vi "Send Message_test.vi"(2 "msj":string, 4 "error in (no error)":errorcluster, 5 "Process":i32, 6 "List of process":string[][](array[string]), 7 "Send msj":bool) -> (0 "error out":errorcluster)   [LabVIEW 2022 SP3]
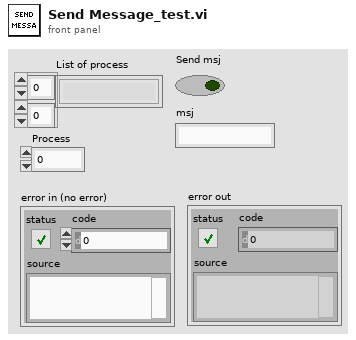
[diagram p1: front panel]
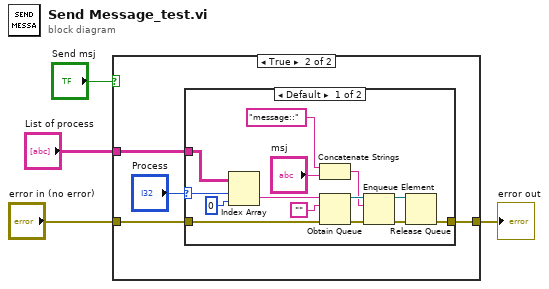
[diagram p0: block diagram]
diagram:
  n1 = case shown="True" "Send msj" {
    tunnel: "List of process" -> [_ w8]
    tunnel: "error in (no error)" -> [w5 w7]
    tunnel: [w5 w6] -> w1
    frame False {
    }
    frame True {
      n2 = case shown="Default" "Process" {
        selector: "Process" -> [w21 _]
        tunnel: w8 -> [w23 _]
        tunnel: w7 -> [w11 w24]
        tunnel: [w10 w24] -> w6
        frame Default {
          n3 = Index Array(array=w23, index (row)=w21, index (col)=0 ("disabled index (col)")) -> (element=w20:string)
          n4 = Concatenate Strings("message::", "msj") -> (w14:string)
          n5 = Obtain Queue(name (unnamed)=w20, element data type="", error in (no error)=w11) -> (queue out=w18:refnum<queue>, error out=w17:errorcluster)  [unwired: 2 in, 1 out]
          n6 = Enqueue Element(queue=w18, element=w14, error in (no error)=w17) -> (queue out=w13:refnum<queue>, error out=w12:errorcluster)  [unwired: 1 in, 1 out]
          n7 = Release Queue(queue=w13, error in (no error)=w12) -> (error out=w10:errorcluster)  [unwired: 1 in, 2 out]
        }
        frame ..-1 {
        }
      }
    }
  }
  "error out" <- w1
